vi "Capture@LoadFiles2Imaq__Parameter.vi"(1 "ParamterIn":string) -> (0 "ParamterOut":string)   [LabVIEW 2020]
uses:
  MainFrame/Global.vi
  <vilib>/vision/NI_Vision_Development_Module.lvlib
panel:
  out "filenames":string[](array[string])
  out "Image":T1(plugin-control)
  in  "Preview":bool
  in  "FilePattern":string(combo)
  in  "FilePath":string(combo)
  in  "Imaq":string(combo)
  in  "Confirm":bool
  # "Capture@LoadFiles2Imaq $Imaq,$FilePattern\n$MainARCOSDir\\Picture"
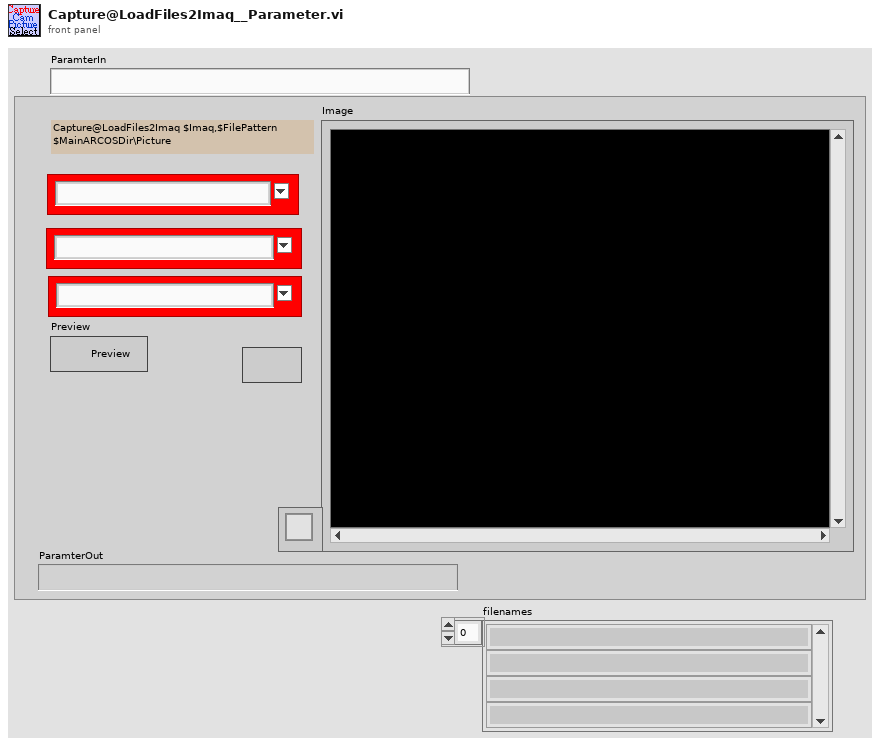
[diagram p1: front panel]
types:
  T1 = typedef "IMAQ Image.ctl" = refnum<image>
  T2 = enum16{"Get", "Get&Index+1", "Insert", "Init", "Clear", "SetIndex"}
  T3 = cluster{"Browser Size":cluster{"X":i32, "Y":i32}, "Images per Line":i32, "Background Color":u32, "Frame Size":i32, "Frame Style":u16}
  T4 = typedef "Image Type" = u32
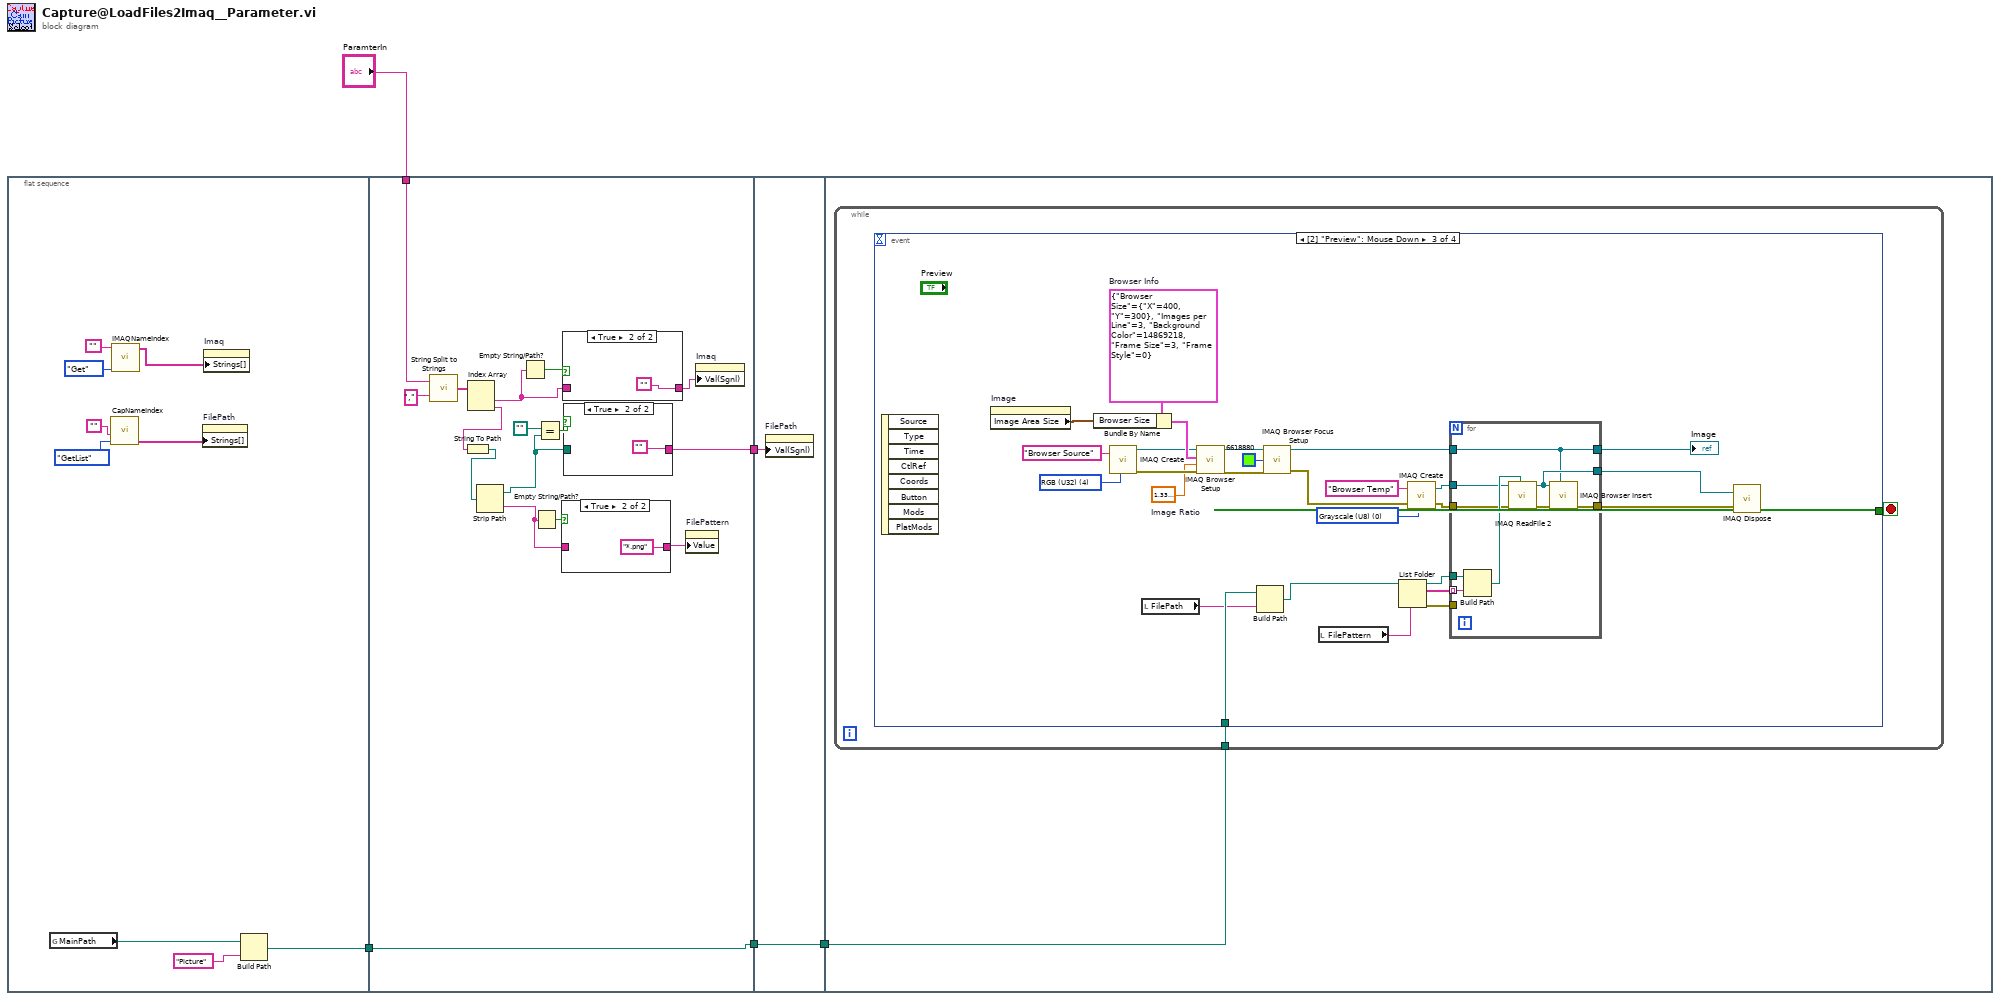
[diagram p0: block diagram]
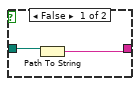
[diagram p3: hidden frame]
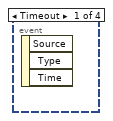
[diagram p5: hidden frame]
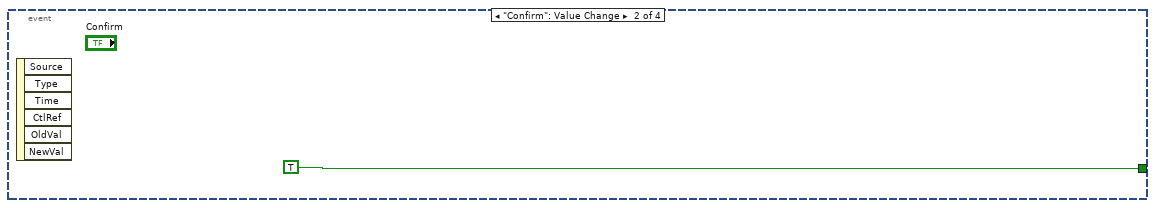
[diagram p6: hidden frame]
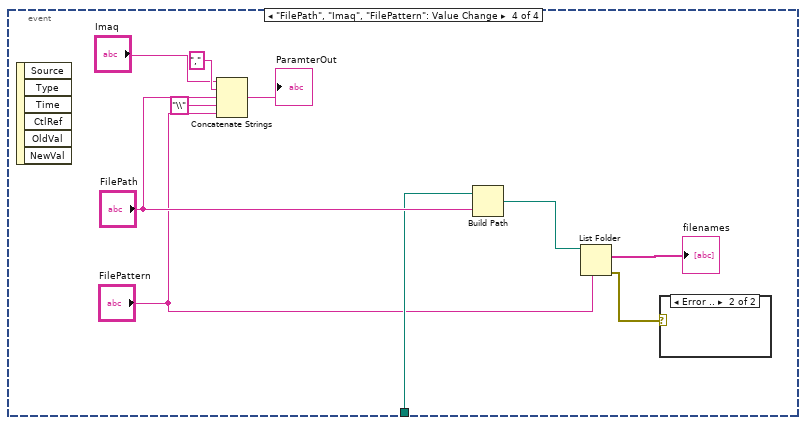
[diagram p7: hidden frame]
diagram:
  n1 = flat-sequence {
    tunnel: [w11] -> w2
    tunnel: "ParamterIn" -> [w28]
    tunnel: [w26] -> w3
    tunnel: w2 -> [w26]
    tunnel: [w25] -> w1
    tunnel: [w39] -> w4
    tunnel: w3 -> [w39]
    tunnel: w1 -> [w38]
    tunnel: w4 -> [w40]
    frame #0 {
      n2 = global read "Global.vi" "MainPath"() -> (w6:path)
      n3 = call "CapNameIndex.vi"("OP"=enum16{"AddCam", "GetIndex", "Init", "GetList"}."GetList", "CamName"="") -> ("DeviceList"=w7:string[])  [unwired: 2 in, 3 out]
      n4 = call "IMAQNameIndex.vi"("OP"=T2."Get", "IMAQName"="") -> ("IMAQNameList"=w8:string[])  [unwired: 2 in, 7 out]
      n5 = property on="FilePath" class="CmbBox"("Strings[]"=w7) -> ()  [unwired: 2 in, 2 out]
      n6 = property on="Imaq" class="CmbBox"("Strings[]"=w8) -> ()  [unwired: 2 in, 2 out]
      n7 = Build Path(base path=w6, name or relative path="Picture") -> (appended path=w11:path)
    }
    frame #1 {
      n8 = call "String Split to Strings.vi"("search string/char (-)"=",", "String"=w28) -> ("Array"=w30:string[])
      n9 = Index Array(array=w30) -> (element #1=w22:string, element #2=w20:string)  [unwired: 2 in]
      n10 = String To Path(string=w20) -> (path=w19:path)
      n11 = Strip Path(path=w19) -> (stripped path=w16:path, name=w18:string)
      n12 = Empty String/Path?(string/path=w22) -> (empty?=w27:bool)
      n13 = Empty String/Path?(string/path=w18) -> (empty?=w24:bool)
      n14 = Equal?(x=path "", y=w16) -> (x = y?=w15:bool)
      n15 = case shown="True" w24 {
        tunnel: [w31 "*.png"] -> w23
        tunnel: w18 -> [w31 _]
        frame False {
        }
        frame True {
        }
      }
      n16 = case shown="True" w27 {
        tunnel: w22 -> [w36 _]
        tunnel: [w36 ""] -> w21
        frame False {
        }
        frame True {
        }
      }
      n17 = case shown="True" w15 {
        tunnel: [w33 ""] -> w25
        tunnel: w16 -> [w34 _]
        frame False {
          n18 = Path To String(path=w34) -> (string=w33:string)
        }
        frame True {
        }
      }
      n19 = property on="FilePattern" class="CmbBox"("Value"=w23) -> ()  [unwired: 2 in, 2 out]
      n20 = property on="Imaq" class="CmbBox"("Val(Sgnl)"=w21) -> ()  [unwired: 2 in, 2 out]
    }
    frame #2 {
      n21 = property on="FilePath" class="CmbBox"("Val(Sgnl)"=w38) -> ()  [unwired: 2 in, 2 out]
    }
    frame #3 {
      n22 = while {
        tunnel: w40 -> [w41]
        stop <- w42 stop-if-true
        n23 = event shown="[2] \"Preview\": Mouse Down" {
          selector: _ -> [_ _ _ _]
          dyn-events: _ -> [_ _ _ _]
          timeout: _ -> [_ _ _ _]
          tunnel: [_ TRUE _ _] -> w42
          tunnel: w41 -> [_ _ w46 w83]
          event Timeout {
            n24 = event-data() -> ()  [unwired: 1 in, 3 out]
          }
          event "Confirm": Value Change {
            n25 = event-data() -> ()  [unwired: 1 in, 6 out]
          }
          event "Preview": Mouse Down {
            w48 = sgl 1.33  # Image Ratio
            w66 = T3 {"Browser Size"={"X"=400, "Y"=300}, "Images per Line"=3, "Background Color"=14869218, "Frame Size"=3, "Frame Style"=0}  # Browser Info
            w57 = T4 0 items=["Grayscale (U8)", "Grayscale (I16)", "Grayscale (SGL)", "Complex (CSG)", "RGB (U32)", "HSL (U32)", "RGB (U64)", "Grayscale (U16)"] ("Image Type")
            w55 = T4 4 items=["Grayscale (U8)", "Grayscale (I16)", "Grayscale (SGL)", "Complex (CSG)", "RGB (U32)", "HSL (U32)", "RGB (U64)", "Grayscale (U16)"] ("Image Type")
            n26 = event-data() -> ()  [unwired: 1 in, 8 out]
            n27 = property on="Image" class="ImageControl"() -> ("Image Area Size"=w67:cluster{"Width":u32, "Height":u32})  [unwired: 2 in, 2 out]
            n28 = Bundle By Name(cluster=w66, "Browser Size"=w67) -> (w68:T3)
            n29 = call "IMAQ Create"("Image Name"="Browser Source", "Image Type"=w55) -> ("New Image"=w53:T1, "error out"=w54:errorcluster)  [unwired: 3 in]
            n30 = local read "FilePath"() -> (w45:string)
            n31 = call "IMAQ Browser Setup"("error in (no error)"=w54, "Image Ratio"=w48, "Browser Info"=w68, "Image In"=w53) -> ("error out"=w62:errorcluster, "Image Browser Out"=w61:T1)  [unwired: 2 out]
            n32 = Build Path(base path=w46, name or relative path=w45) -> (appended path=w44:path)
            n33 = call "IMAQ Browser Focus Setup"("error in (no error)"=w62, "Focus Color"=u32 6618880, "Image Browser In"=w61) -> ("error out"=w64:errorcluster, "Image Browser Out"=w63:T1)  [unwired: 1 in]
            n34 = local read "FilePattern"() -> (w47:string)
            n35 = List Folder(path=w44, pattern=w47) -> (path out=w51:path, filenames=w52:string[], error out=w69:errorcluster)  [unwired: 2 in, 1 out]
            n36 = call "IMAQ Create"("Image Name"="Browser Temp", "Image Type"=w57, "error in (no error)"=w64) -> ("New Image"=w59:T1, "error out"=w49:errorcluster)  [unwired: 2 in]
            n37 = for {
              tunnel: w63 -> [w71]
              tunnel: w51 -> [w79]
              tunnel: w52 -> [w76] mode=indexing
              tunnel: w49 -> [w75]
              tunnel: [w74] -> w50
              tunnel: [w71] -> w70
              tunnel: w59 -> [w73]
              tunnel: [w72] -> w60
              tunnel: w69 -> [_]
              n38 = Build Path(base path=w79, name or relative path=w76) -> (appended path=w78:path)
              n39 = call "IMAQ ReadFile 2"("File Path"=w78, "error in (no error)"=w75, "Image"=w73) -> ("error out"=w77:errorcluster, "Image Out"=w72:T1)  [unwired: 4 in, 3 out]
              n40 = call "IMAQ Browser Insert"("Image Browser In"=w71, "error in (no error)"=w77, "Image to Add"=w72) -> ("error out"=w74:errorcluster)  [unwired: 4 in, 4 out]
            }
            "Image" <- w70
            n41 = call "IMAQ Dispose"("Image"=w60, "error in (no error)"=w50) -> ()  [unwired: 4 in, 1 out]
          }
          event "FilePath", "Imaq", "FilePattern": Value Change {
            n42 = event-data() -> ()  [unwired: 1 in, 6 out]
            n43 = Concatenate Strings("Imaq", "," ("string"), "FilePath", "\\" ("string"), "FilePattern") -> (→"ParamterOut":string)
            n44 = Build Path(base path=w83, name or relative path="FilePath") -> (appended path=w82:path)
            n45 = List Folder(path=w82, pattern="FilePattern") -> (filenames=→"filenames":string[], error out=w84:errorcluster)  [unwired: 2 in, 2 out]
            n46 = case shown="Error .." w84 {
              frame No Error {
              }
              frame Error {
              }
            }
          }
        }
      }
    }
  }
